vi "DBM_InsertRow.vi"(8 "error in (no error)":errorcluster, 9 "Offset(s)":dbl, 10 "IsStart?":bool, 11 "DBManager in":refnum<class "DBManager.lvclass">) -> (0 "error out":errorcluster, 3 "DBManager out":refnum<class "DBManager.lvclass">)   [LabVIEW 2015, in "DBManager.lvclass"]
uses:
  DBManager.lvclass
  DBManager.lvclass/DBManager.ctl
  <vilib>/drjdpowell/SQLite Library/SQL Statement/SQL Statement.lvclass/SQL Statement.ctl
  <vilib>/drjdpowell/SQLite Library/SQL Statement/Bind Timestamp (Real).vi
  <vilib>/drjdpowell/SQLite Library/SQL Statement/Bind Integer.vi
  <vilib>/drjdpowell/SQLite Library/SQL Statement/Step.vi
  <vilib>/drjdpowell/SQLite Library/SQL Statement/Bind Real.vi
  <vilib>/drjdpowell/SQLite Library/SQL Statement/Error Message.vi
  <vilib>/drjdpowell/SQLite Library/SQL Connection/Connection.lvclass
  <vilib>/drjdpowell/SQLite Library/SQL Statement/SQL Statement.lvclass
  <vilib>/drjdpowell/SQLite Library/Transaction Helpers/Transaction.lvlib
panel:
  # "Connector Pane"
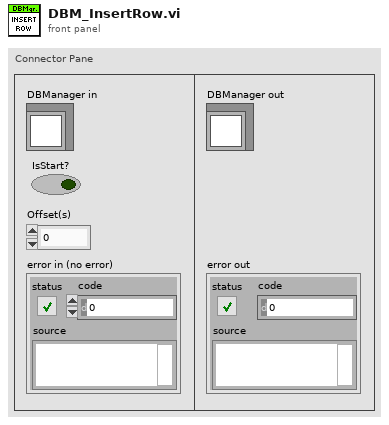
[diagram p1: front panel]
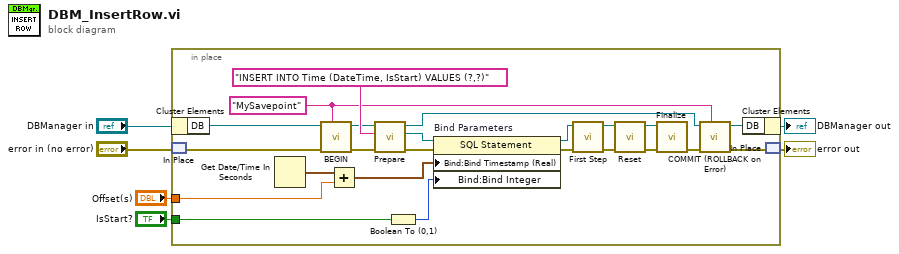
[diagram p0: block diagram]
diagram:
  n1 = in-place {
    in-place-border: "IsStart?" -> [w9]
    in-place-border: "Offset(s)" -> [w7]
    w22 = "MySavepoint" ("Savepoint name")
    n2 = in-place-cluster #1("DBManager in") -> ("DB"=w18:refnum<class "Connection.lvclass">)
    n3 = in-place-match #2("error in (no error)") -> (w19:errorcluster)
    n4 = Get Date/Time In Seconds() -> (seconds since 1Jan1904=w15:timestamp)
    n5 = call <vilib>:"BEGIN.vi"("Savepoint name"=w22, "error in (no error)"=w19, "Connection in"=w18) -> ("error out"=w23:errorcluster, "Connection out"=w24:refnum<class "Connection.lvclass">)  [unwired: 7 in]
    n6 = Add(x=w15, y=w7) -> (x+y=w8:timestamp)
    n7 = call <vilib>:"Prepare.vi"("error in (no error)"=w23, "SQL"="INSERT INTO Time (DateTime, IsStart) VALUES (?,?)" ("INSERT statement"), "SQLite Connection in"=w24) -> ("error out"=w28:errorcluster, "SQL Statement out"=w29:refnum<class "SQL Statement.lvclass">, "SQLite Connection out"=w21:refnum<class "Connection.lvclass">)  [unwired: 4 in, 2 out]
    n8 = Boolean To (0,1)(Boolean=w9) -> (0, 1=w14:i16)
    n9 = property on="Bind Parameters" class="SQL Statement"(reference=w29, error in=w28, "Bind:Bind Timestamp (Real)"=w8, "Bind:Bind Integer"=w14) -> (reference out=w13:refnum<class "SQL Statement.lvclass">, error out=w12:errorcluster)
    n10 = call <vilib>:"First Step.vi"("error in (no error)"=w12, "SQL Statement in"=w13) -> ("error out"=w11:errorcluster, "SQL Statement out"=w10:refnum<class "SQL Statement.lvclass">)  [unwired: 7 in, 1 out]
    n11 = call <vilib>:"Reset.vi"("error in (no error)"=w11, "SQL Statement in"=w10) -> ("error out"=w25:errorcluster, "SQL Statement out"=w26:refnum<class "SQL Statement.lvclass">)  [unwired: 8 in]
    n12 = call <vilib>:"Finalize.vi"("error in (no error)"=w25, "SQL Statement in"=w26) -> ("error out"=w20:errorcluster)  [unwired: 9 in]
    n13 = call <vilib>:"COMMIT (ROLLBACK on Error).vi"("Savepoint name"=w22, "error in (no error)"=w20, "Connection in"=w21) -> ("error out"=w17:errorcluster, "Connection out"=w16:refnum<class "Connection.lvclass">)  [unwired: 7 in]
    n14 = in-place-cluster #1("DB"=w16) -> (→"DBManager out":refnum<class "DBManager.lvclass">)
    n15 = in-place-match #2(w17) -> (→"error out":errorcluster)
  }
